vi "table-test.vi"() -> ()   [LabVIEW 2014]
uses:
  <vilib>/Utility/miscctls.llb/LVBoundsTypeDef.ctl
panel:
  in  "stop":bool
  in  "Omicron":bool
  in  "Ageing - Cycle Pattern":string[][](table) caption="Subcycle pattern"
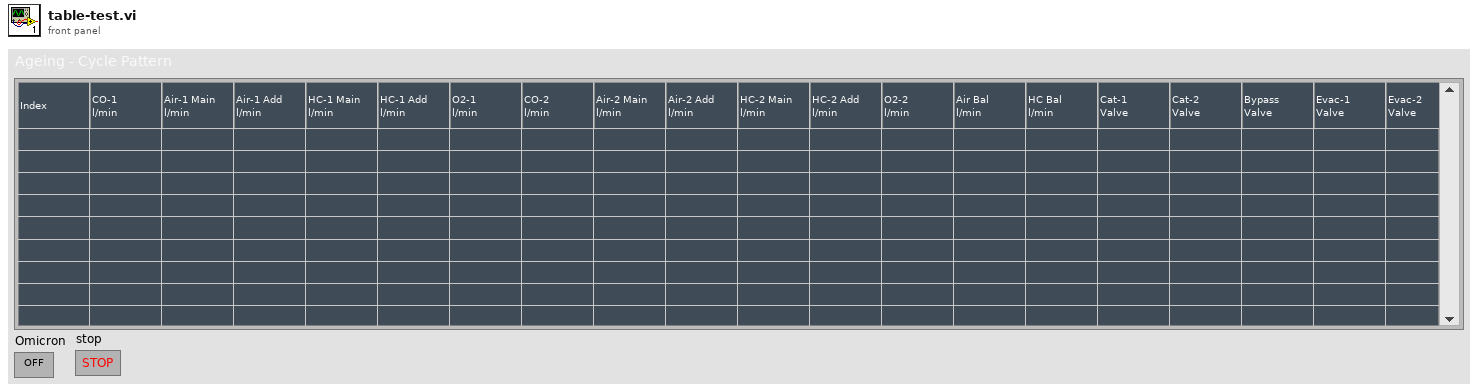
[diagram p1: front panel]
types:
  T1 = typedef "LVBoundsTypeDef.ctl" = cluster{"Width":u32, "Height":u32}
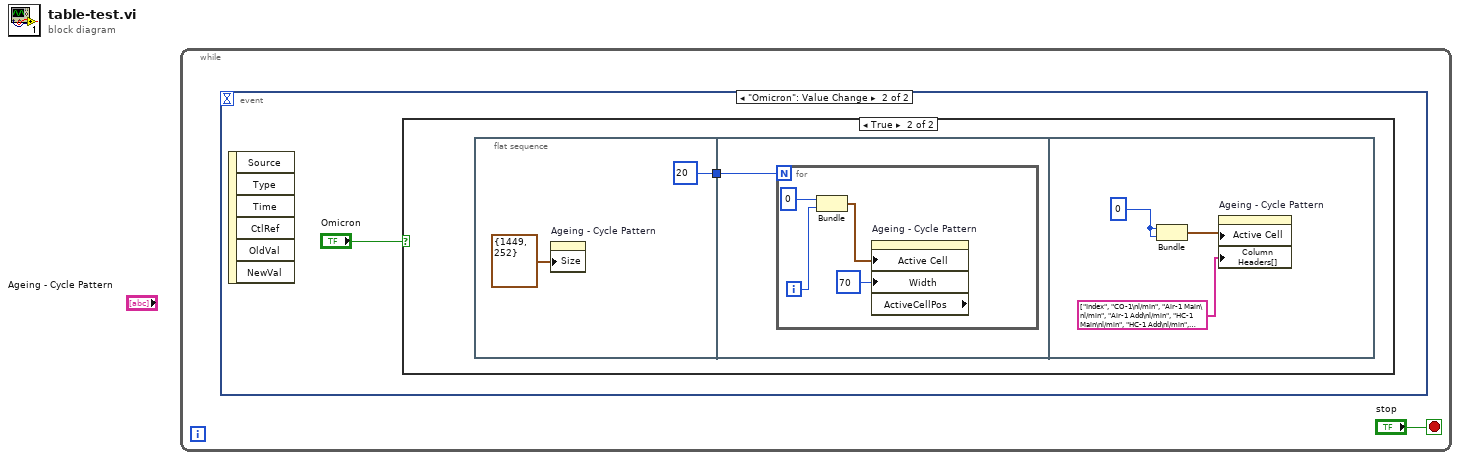
[diagram p0: block diagram]
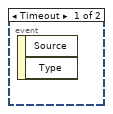
[diagram p2: hidden frame]
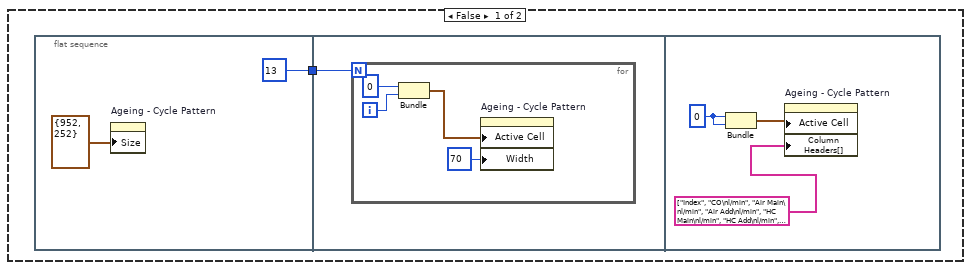
[diagram p3: hidden frame]
diagram:
  n1 = while {
    stop <- "stop" stop-if-true
    n2 = event shown="[1] \"Omicron\": Value Change" {
      selector: _ -> [_ _]
      dyn-events: _ -> [_ _]
      timeout: _ -> [_ _]
      event Timeout {
        n3 = event-data() -> ()  [unwired: 1 in, 2 out]
      }
      event "Omicron": Value Change {
        n4 = event-data() -> ()  [unwired: 1 in, 6 out]
        n5 = case shown="True" "Omicron" {
          frame False {
            n6 = flat-sequence {
              tunnel: [13] -> w3
              tunnel: w3 -> [w6]
              frame #0 {
                n7 = property on="Ageing - Cycle Pattern" class="Tbl (strict)"("Size"=T1 {"Width"=952, "Height"=252}) -> ()  [unwired: 2 in, 2 out]
              }
              frame #1 {
                n8 = for {
                  N: w6 -> [_]
                  i -> [w8]
                  n9 = Bundle(0, w8) -> (w7:cluster{i32, i32})  [unwired: 1 in]
                  n10 = property on="Ageing - Cycle Pattern" class="Tbl (strict)"("Active Cell"=w7, "Width"=u32 70 ("Active Cell:Cell Size:Width")) -> ()  [unwired: 2 in, 2 out]
                }
              }
              frame #2 {
                w13 = 0
                n11 = Bundle(w13, w13) -> (w12:cluster{i32, i32})  [unwired: 1 in]
                n12 = property on="Ageing - Cycle Pattern" class="Tbl (strict)"("Active Cell"=w12, "Column Headers[]"=string[] ["Index", "CO\nl/min", "Air Main\nl/min", "Air Add\nl/min", "HC Main\nl/min", "HC Add\nl/min", "NO\nl/min", "Air Bal\nl/min", "HC Bal\nl/min", "O2\nl/min", "Pre-Cat\nValve", "Bypass\nValve", "Evac \nValve"] ("Row Header Strings[]")) -> ()  [unwired: 2 in, 2 out]
              }
            }
          }
          frame True {
            n13 = flat-sequence {
              tunnel: [20] -> w14
              tunnel: w14 -> [w17]
              frame #0 {
                n14 = property on="Ageing - Cycle Pattern" class="Tbl (strict)"("Size"=T1 {"Width"=1449, "Height"=252}) -> ()  [unwired: 2 in, 2 out]
              }
              frame #1 {
                n15 = for {
                  N: w17 -> [_]
                  i -> [w19]
                  n16 = Bundle(0, w19) -> (w18:cluster{i32, i32})  [unwired: 1 in]
                  n17 = property on="Ageing - Cycle Pattern" class="Tbl (strict)" props=["Active Cell", "Width", "ActiveCellPos"]("Active Cell"=w18, "Width"=u32 70 ("Active Cell:Cell Size:Width")) -> ()  [unwired: 2 in, 3 out]
                }
              }
              frame #2 {
                w23 = 0
                n18 = Bundle(w23, w23) -> (w24:cluster{i32, i32})  [unwired: 1 in]
                n19 = property on="Ageing - Cycle Pattern" class="Tbl (strict)"("Active Cell"=w24, "Column Headers[]"=string[] ["Index", "CO-1\nl/min", "Air-1 Main\nl/min", "Air-1 Add\nl/min", "HC-1 Main\nl/min", "HC-1 Add\nl/min", "O2-1\nl/min", "CO-2\nl/min", "Air-2 Main\nl/min", "Air-2 Add\nl/min", "HC-2 Main\nl/min", "HC-2 Add\nl/min", "O2-2\nl/min", "Air Bal\nl/min", "HC Bal\nl/min", "Cat-1\nValve", "Cat-2\nValve", "Bypass\nValve", "Evac-1\nValve", "Evac-2\nValve"] ("Row Header Strings[]")) -> ()  [unwired: 2 in, 2 out]
              }
            }
          }
        }
      }
    }
  }
